vi "GetShifterState.vi"(7 "Sensor Failure":bool, 9 "Low Gear Sensor":bool, 10 "High Gear Sensor":bool) -> (2 "Actual Shifter State":T1(ring))   [LabVIEW 2019]
doc: "This VI interpretes the values from two photointerruptor sensors to determine the true current state of the drive module shifting mechanism."
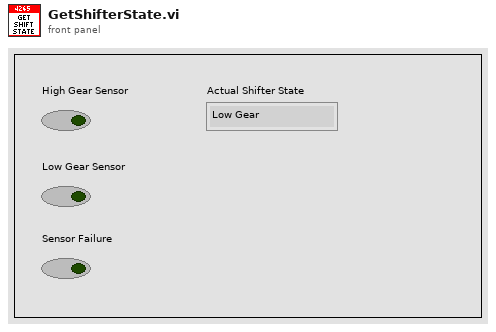
[diagram p1: front panel]
types:
  T1 = enum16{"Low Gear", "High Gear", "Transiting", "Unknown"}
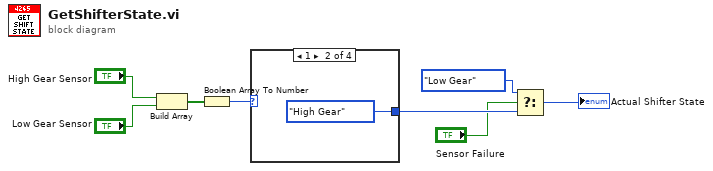
[diagram p0: block diagram]
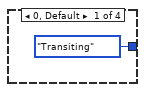
[diagram p2: hidden frame]
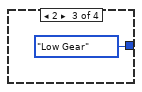
[diagram p3: hidden frame]
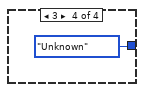
[diagram p4: hidden frame]
diagram:
  n1 = Build Array("High Gear Sensor", "Low Gear Sensor") -> (w6:bool[])
  n2 = Boolean Array To Number(Boolean array=w6) -> (number=w5:u32)
  n3 = case shown="1" w5 {
    tunnel: [T1."Transiting" ("Actual_Shifter_State") T1."High Gear" ("Actual_Shifter_State") T1."Low Gear" ("Actual_Shifter_State") T1."Unknown" ("Actual_Shifter_State")] -> w4
    frame 0, Default {
    }
    frame 1 {
    }
    frame 2 {
    }
    frame 3 {
    }
  }
  n4 = Select(t=T1."Low Gear", s="Sensor Failure", f=w4) -> (s? t:f=→"Actual Shifter State":T1)
